vi "Initilaize Sinks.vi"(8 "error in (no error)":errorcluster, 11 "Example Source in":refnum<class "Example Source.lvclass">) -> (0 "error out":errorcluster, 3 "Example Source out":refnum<class "Example Source.lvclass">)   [LabVIEW 2016, in "Example Source.lvlib" / "Example Source.lvclass"]
uses:
  Example Source.lvclass
  C:/Projects/Shared Libraries/Event Actors/Event Source/Event Source.lvclass
  Alternative Example Sink/Example Sink/Alternative Example Sink.lvclass
  C:/Projects/Shared Libraries/Event Actors/Event Sink/Event Sink.lvclass
  Event Sink/Event Sink.lvclass/Event Sink.ctl
  Event Sink/properties/Write Name.vi
  Event Source/Event Source.lvclass
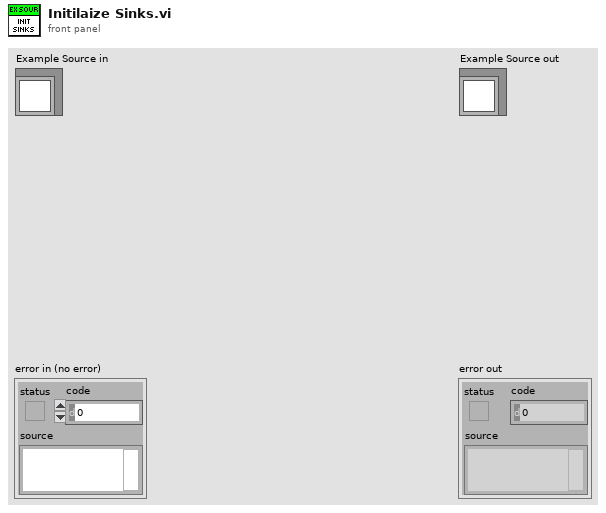
[diagram p1: front panel]
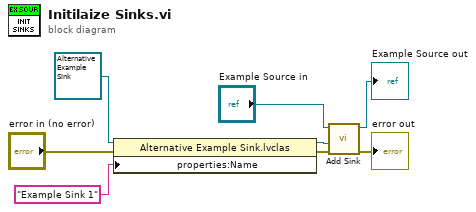
[diagram p0: block diagram]
diagram:
  n1 = property class="Alternative Example Sink.lvclas"(reference=refnum<class "Alternative Example Sink.lvclass"> refnum ("Alternative Example Sink.lvlib:Alternative Example Sink.lvclass"), error in="error in (no error)", "properties:Name"="Example Sink 1" ("Debug Alias")) -> (reference out=w4:refnum<class "Alternative Example Sink.lvclass">, error out=w1:errorcluster)
  n2 = call "Add Sink.vi"("error in (no error)"=w1, "Sink Actor"=w4, "Event Source in"="Example Source in") -> ("error out"=→"error out":errorcluster, "Event Source out"=→"Example Source out":refnum<class "Example Source.lvclass">)  [unwired: 7 in]
